vi "Error Handling.vi"(8 "error in (no error)":errorcluster, 10 "HTTP headers":T1, 11 "HTTP status code":string) -> (0 "error out":errorcluster)   [LabVIEW 2018, in "InfluxDB Client.lvlib" / "Client.lvclass"]
uses:
  Client.lvclass
  <userlib>/_OpenG.lib/dictionary/dictionary.llb/Dictionary Object RefNum__ogtk.ctl
  <userlib>/_OpenG.lib/dictionary/dictionary.llb/Dictionary Object RefNum - Enum__ogtk.ctl
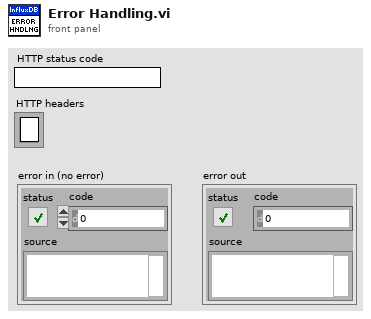
[diagram p1: front panel]
types:
  T1 = typedef "Dictionary Object RefNum__ogtk.ctl" = refnum<k1>
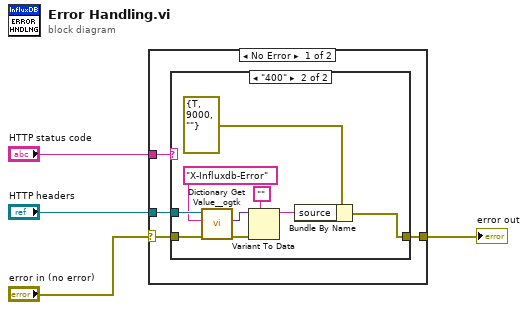
[diagram p0: block diagram]
diagram:
  n1 = case shown="No Error" "error in (no error)" {
    selector: "error in (no error)" -> [w5 w19]
    tunnel: "HTTP headers" -> [w8 _]
    tunnel: [w7 w19] -> w3
    tunnel: "HTTP status code" -> [w6 _]
    frame No Error {
      n2 = case shown="\"400\"" w6 {
        tunnel: w5 -> [w9 w10]
        tunnel: [w9 w13] -> w7
        tunnel: w8 -> [_ w18]
        frame "200", Default {
        }
        frame "400" {
          n3 = call <userlib>:"Dictionary Get Value__ogtk.vi"("error in"=w10, "key"="X-Influxdb-Error", "dictionary"=w18) -> ("error out"=w11:errorcluster, "value"=w16:variant)  [unwired: 5 in, 2 out]
          n4 = Variant To Data(error in=w11, type="", Variant=w16) -> (data=w14:string)  [unwired: 1 out]
          n5 = Bundle By Name(cluster=errorcluster {"status"=TRUE, "code"=9000, "source"=""} ("error constant"), "source"=w14) -> (w13:errorcluster)
        }
      }
    }
    frame Error {
    }
  }
  "error out" <- w3
